vi "Report formate.vi"(8 "error in (no error)":errorcluster, 11 "template (empty)":path=path "G:/Magnetic Mareli UM/MM_UM/Report/Template.doc") -> (0 "error out":errorcluster)   [LabVIEW 2015]
uses:
  <vilib>/Utility/NIReport.llb/Append Report Text (str wrap).vi
  <vilib>/Utility/NIReport.llb/Append Text Table to Report (wrap).vi
  <vilib>/Utility/NIReport.llb/NI_report.lvclass
  <vilib>/Utility/NIReport.llb/Word/NI_Word.lvclass
panel:
  in  "text data 2":string[][](array[string])
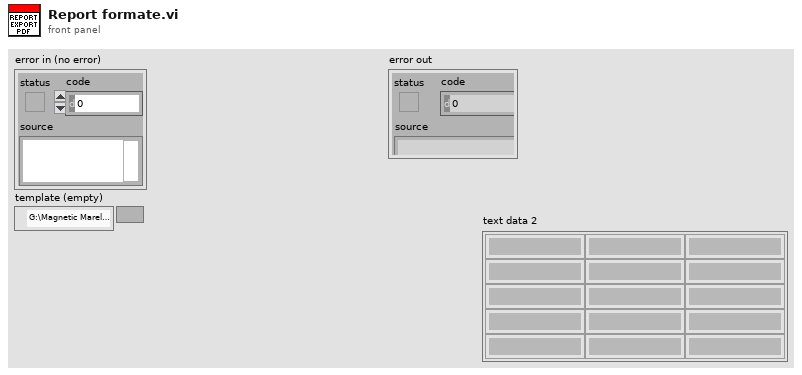
[diagram p1: front panel]
types:
  T1 = cluster{"position (excel)":cluster{"row":i32, "column":i32}, "name (excel)":string, "bookmark (word)":string}
  T2 = enum16{"Standard Report", "HTML", "Word", "Excel"}
  T3 = enum16{"maximized", "minimized", "normal", "no change"}
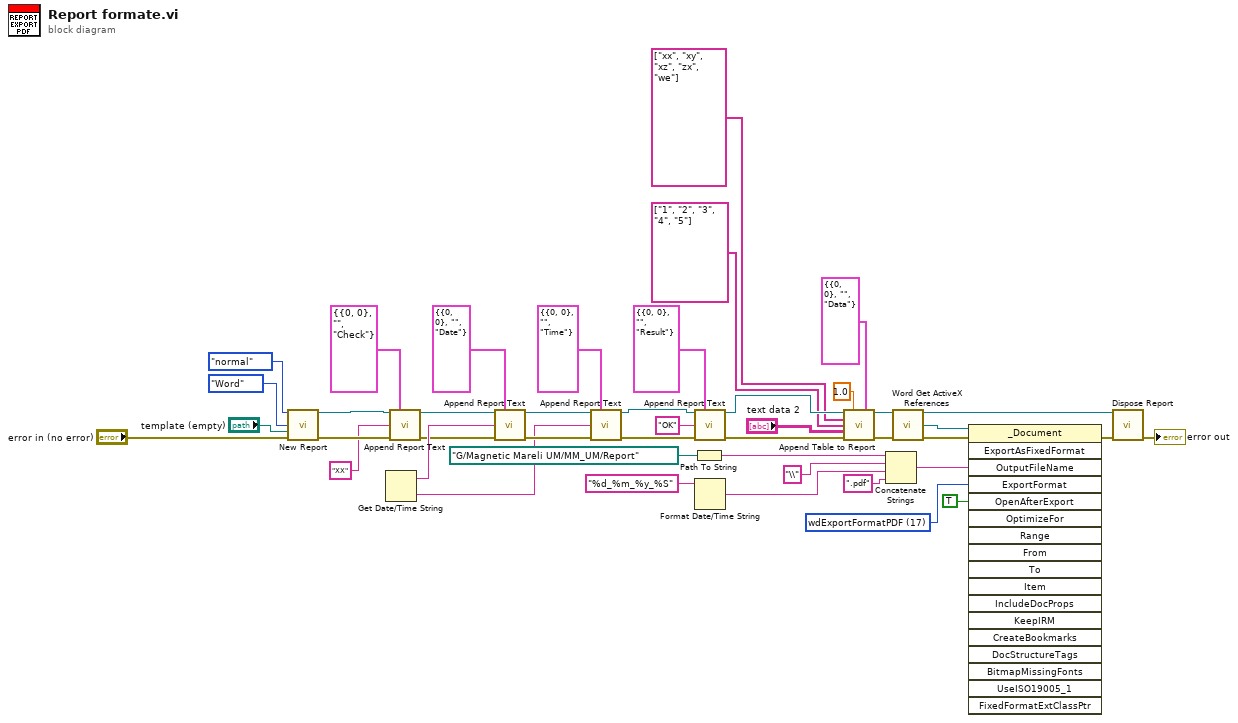
[diagram p0: block diagram]
diagram:
  w31 = 17 items=["wdExportFormatPDF"=17, "wdExportFormatXPS"=18] ("ExportFormat")
  n1 = call <vilib>:"New Report.vi"("window state (normal)"=T3."normal", "report type"=T2."Word", "template (empty)"="template (empty)", "error in (no error)"="error in (no error)") -> ("report out"=w33:refnum<class "NI_report.lvclass">, "error out"=w36:errorcluster)  [unwired: 10 in]
  n2 = Get Date/Time String() -> (date string=w13:string, time string=w12:string)  [unwired: 3 in]
  n3 = call-poly <vilib>:"Append Report Text.vi"("report in"=w33, "MS Office parameters"=T1 {"position (excel)"={"row"=0, "column"=0}, "name (excel)"="", "bookmark (word)"="Check"}, "text"="XX", "error in (no error)"=w36) -> ("report out"=w6:refnum<class "NI_report.lvclass">, "error out"=w7:errorcluster)  [unwired: 8 in, 2 out]
  n4 = call-poly <vilib>:"Append Report Text.vi"("report in"=w6, "MS Office parameters"=T1 {"position (excel)"={"row"=0, "column"=0}, "name (excel)"="", "bookmark (word)"="Date"}, "text"=w13, "error in (no error)"=w7) -> ("report out"=w17:refnum<class "NI_report.lvclass">, "error out"=w16:errorcluster)  [unwired: 8 in, 2 out]
  n5 = call-poly <vilib>:"Append Report Text.vi"("report in"=w17, "MS Office parameters"=T1 {"position (excel)"={"row"=0, "column"=0}, "name (excel)"="", "bookmark (word)"="Time"}, "text"=w12, "error in (no error)"=w16) -> ("report out"=w15:refnum<class "NI_report.lvclass">, "error out"=w14:errorcluster)  [unwired: 8 in, 2 out]
  n6 = Path To String(path=path "G:/Magnetic Mareli UM/MM_UM/Report") -> (string=w23:string)
  n7 = call-poly <vilib>:"Append Report Text.vi"("report in"=w15, "MS Office parameters"=T1 {"position (excel)"={"row"=0, "column"=0}, "name (excel)"="", "bookmark (word)"="Result"}, "text"="OK", "error in (no error)"=w14) -> ("report out"=w35:refnum<class "NI_report.lvclass">, "error out"=w34:errorcluster)  [unwired: 8 in, 2 out]
  n8 = Format Date/Time String(time format string (%c)="%d_%m_%y_%S") -> (date/time string=w20:string)  [unwired: 2 in]
  n9 = call-poly <vilib>:"Append Table to Report.vi"("report in"=w35, "column width (1)"=1.0, "MS Office parameters"=T1 {"position (excel)"={"row"=0, "column"=0}, "name (excel)"="", "bookmark (word)"="Data"}, "column headers"=string[] ["xx", "xy", "xz", "zx", "we"] ("row headers"), "row headers"=string[] ["1", "2", "3", "4", "5"] ("column headers"), "text data"="text data 2", "error in (no error)"=w34) -> ("report out"=w27:refnum<class "NI_report.lvclass">, "error out"=w26:errorcluster)  [unwired: 5 in, 2 out]
  n10 = Concatenate Strings(w23, "\\" ("string"), w20, ".pdf" ("string")) -> (w22:string)
  n11 = call <vilib>:"Word Get ActiveX References.vi"("report in"=w27, "error in (no error)"=w26) -> ("report out"=w39:refnum<class "NI_report.lvclass">, "Word._Document"=w32:refnum<k7>, "error out"=w29:errorcluster)  [unwired: 7 in, 4 out]
  n12 = invoke class="_Document" method="ExportAsFixedFormat"(reference=w32, error in=w29, "OutputFileName"=w22, "ExportFormat"=w31, "OpenAfterExport"=TRUE) -> (error out=w28:errorcluster)  [unwired: 13 in, 17 out]
  n13 = call-dynamic "Dispose Report.vi"("report in"=w39, "error in (no error)"=w28) -> ("error out"=→"error out":errorcluster)  [unwired: 13 in]
